vi "Write.vi"(8 "error in":errorcluster, 10 "CAN Message":T1 {"MSG type" format="%x"; "ID" format="%.0x"}, 11 "ICAN in":refnum<class "ICAN.lvclass">) -> (0 "error out":errorcluster, 3 "ICAN out":refnum<class "ICAN.lvclass">)   [LabVIEW 2024, in "ICAN.lvclass"]
uses:
  ICAN.lvclass
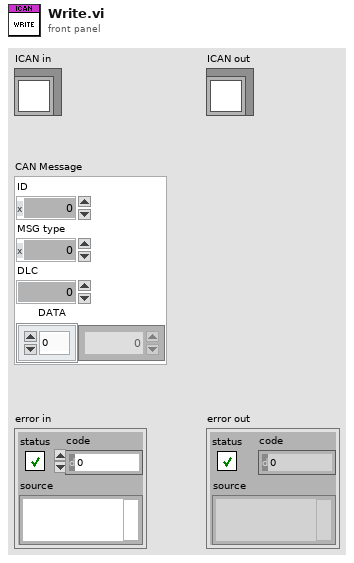
[diagram p1: front panel]
types:
  T1 = cluster{"ID":u32, "MSG type":u8, "DLC":u8, "DATA":u8[]}
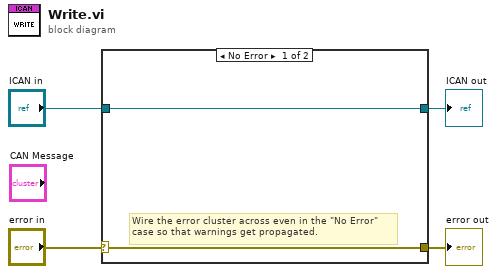
[diagram p0: block diagram]
diagram:
  n1 = case shown="No Error" "error in" {
    selector: "error in" -> [w5 w8]
    tunnel: [w5 w8] -> w3
    tunnel: [w6 w7] -> w1
    tunnel: "ICAN in" -> [w6 w7]
    frame No Error {
      # "Wire the error cluster across even in the \"No Error\"\ncase so that warnings get propagated."
    }
    frame Error {
    }
  }
  "error out" <- w3
  "ICAN out" <- w1
